vi "PH_AxisGUI_NF2.panel.vi"(0 "object ref":refnum<vi>, 5 "error in (no error)":errorcluster) -> (19 "error out":errorcluster)   [LabVIEW 2014, in "PH_AxisGUI_NF2.lvlib"]
doc: "By this VI a ross relais can be monitored and switched. \n\nThe indicators \"CLOSED\", \"OPEN\" and \"SWITCH STATE\" show the value of the Beckhoff-Tag: blue indicates bad tag status reference problems, darkgreen false and lightgreen on. If everything is working fine, \"CLOSED\" and \"SWITCH STATE\" should show the same value, while \"OPEN\" has the opposite value. \n\nThe oval button switches the ross relais. It should be in the same state as the \"SWITCH STATE\" indicator. \n\n\"EXIT\" closes the front panel (GUI), while \"Delete Instance\" disconnects and removes the instance from the PCS.\n\nThis VI has no machine safety relevant logig: there is neither a check of internal conclict nor with other objects, for example conflict with other ross relais. Therefore it must be handled with care and should be operated by well educated operators only. It is forseen exclusively for direct operating and testing of the system. \n\nLicense Agreement for this software:\n\nCopyright (C)\nGesellschaft für Schwerionenforschung, GSI\nPlanckstr. 1\n64291 Darmstadt\nGermany\n\nContact: D.Beck@gsi.de \n\nThis program is free software; you can redistribute it and/or modify it under the terms of the GNU General Public License as published by the Free Software Foundation; either version 2 of the license, or (at your option) any later version.\n\nThis program is distributed in the hope that it will be useful, but WITHOUT ANYW ARRANTY; without even the implied warranty of MERCHANTABILITY or FITNESS FOR A PARTICULAR PURPOSE. See the GNU General License for more details (http://www.gnu.org).\n\nGesellschaft für Schwerionenforschung, GSI\nPlanckstr. 1, 64291 Darmstadt, Germany\nFor all questions and ideas contact: M.Richter@gsi.de, H.Brand@gsi.de or D.Beck@gsi.de.\nLast update: 18-DEC-2002"
uses:
  PH_AxisGUI_NF2.lvlib
  PH_Common/PH_Common.lvlib
  CSMotion/NF87XX/NF87XX.lvlib
  CSCore/CSSystem/CSSystemLib/CSSystemLib.lvlib
  PH_Class/PH_Class.lvlib
panel:
  in  "DOWN":bool caption="? Steps"
  in  "UP":bool caption="? Steps"
  in  "LEFT":bool caption="? Steps"
  in  "RIGHT":bool caption="? Steps"
  in  "Width Axis 2":i32
  in  "Width Axis 1":i32
  out "Instance Status":u32(colorbox)
  in  "Emergeny Stop":bool
  in  "Delete":bool
  # "PCS"
  # "3.40"
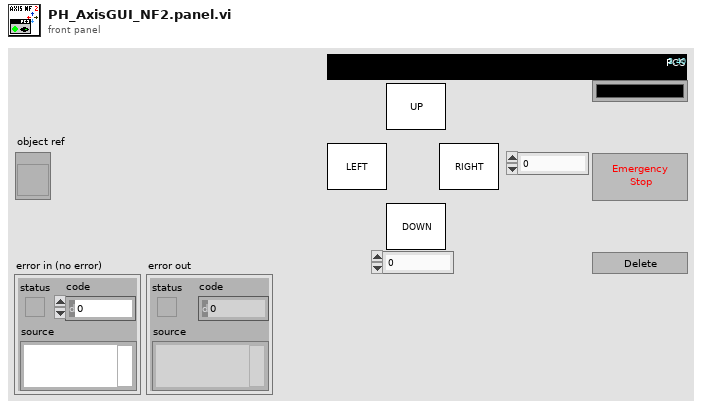
[diagram p1: front panel]
types:
  T1 = typedef "PH_AxisGUI_NF2.lvlib/PH_AxisGUI_NF2.i attribute.ctl" = cluster{"GUI Refs":cluster{"Delete":refnum<vi>, "Instance Status":refnum<vi>, "Width Axis 1":refnum<vi>, "Width Axis 2":refnum<vi>}, "Instance":string, "System":string, "Width Axis 1":i32, "Width Axis 2":i32, "Sign Change Axis 1":bool, "Sign Change Axis 2":bool, "Motor Axis 1":i32, "Motor Axis 2":i32}
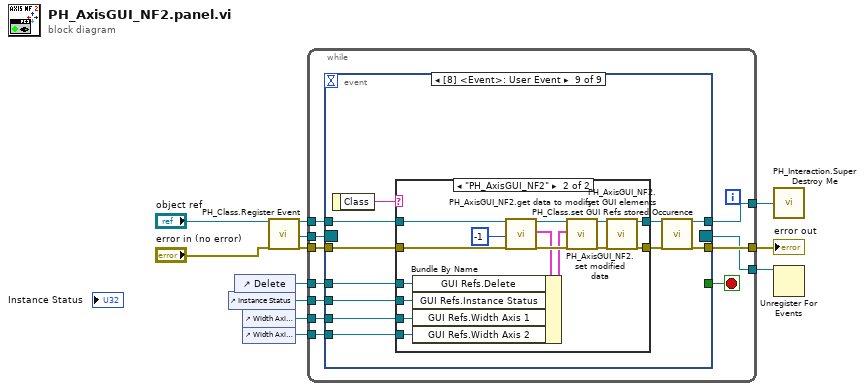
[diagram p0: block diagram]
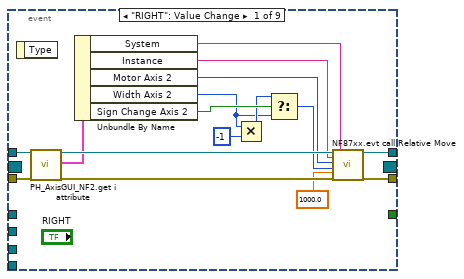
[diagram p2: hidden frame]
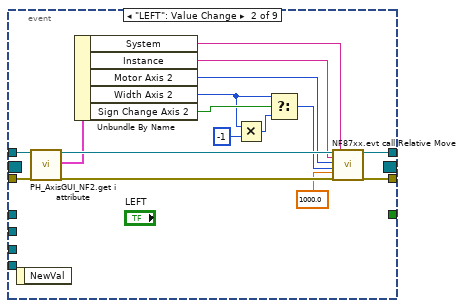
[diagram p3: hidden frame]
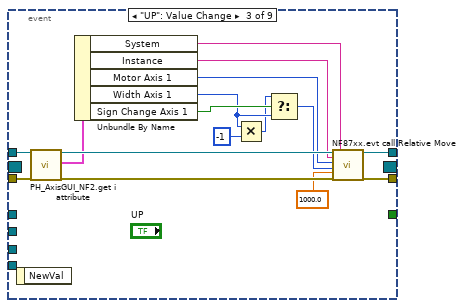
[diagram p4: hidden frame]
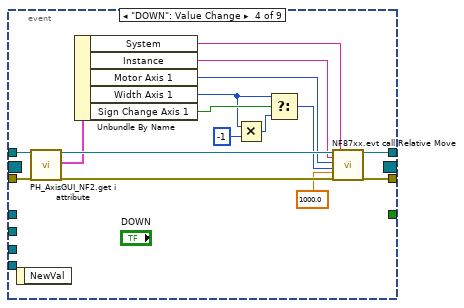
[diagram p5: hidden frame]
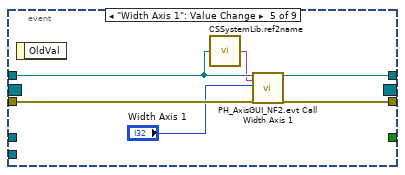
[diagram p6: hidden frame]
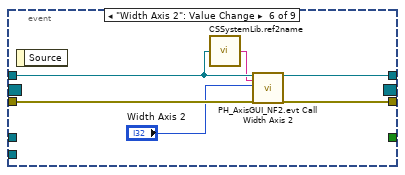
[diagram p7: hidden frame]
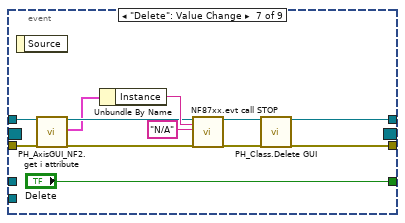
[diagram p8: hidden frame]
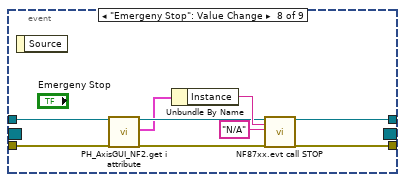
[diagram p9: hidden frame]
diagram:
  n1 = control-ref of="Instance Status"() -> (w3:refnum<vi>)
  n2 = control-ref of="Delete"() -> (w4:refnum<vi>)
  n3 = control-ref of="Width Axis 1"() -> (w2:refnum<vi>)
  n4 = control-ref of="Width Axis 2"() -> (w1:refnum<vi>)
  n5 = call "PH_Class.Register Event.vi"("i ref in"="object ref", "error in (no error)"="error in (no error)") -> ("i ref out"=w10:refnum<vi>, "Event Registration Refnum"=w8:refnum<event-registration>, "error out"=w9:errorcluster)  [unwired: 15 in]
  n6 = while {
    tunnel: w10 -> [w20]
    tunnel: [w19] -> w11
    tunnel: w9 -> [w22]
    tunnel: [w21] -> w12
    tunnel: w8 -> [w18]
    tunnel: [w17] -> w7
    tunnel: w4 -> [w16]
    tunnel: w3 -> [w15]
    tunnel: w2 -> [w14]
    tunnel: w1 -> [w13]
    stop <- w23 stop-if-true
    n7 = event shown="[8] <Event>: User Event" {
      selector: w18 -> [_ _ _ _ _ _ _ _ _]
      dyn-events: [_ _ _ _ _ _ _ _ _] -> w17
      timeout: _ -> [_ _ _ _ _ _ _ _ _]
      tunnel: [_ _ _ _ _ _ "Delete" _ _] -> w23
      tunnel: w20 -> [w37 w53 w69 w85 w89 w96 w106 w116 w131]
      tunnel: w22 -> [w35 w51 w67 w83 w92 w98 w104 w115 w128]
      tunnel: [w38 w54 w70 w86 w91 w97 w100 w112 w126] -> w21
      tunnel: [w39 w55 w71 w87 w93 w99 w101 w113 w129] -> w19
      tunnel: w16 -> [_ _ _ _ _ _ _ _ w124]
      tunnel: w15 -> [_ _ _ _ _ _ _ _ w123]
      tunnel: w14 -> [_ _ _ _ _ _ _ _ w122]
      tunnel: w13 -> [_ _ _ _ _ _ _ _ w121]
      event "RIGHT": Value Change {
        n8 = event-data() -> ()  [unwired: 1 in, 1 out]
        n9 = call "PH_AxisGUI_NF2.get i attribute.vi"("i ref in"=w37, "error in (no error)"=w35) -> ("i ref out"=w36:refnum<vi>, "i attribute"=w33:T1, "error out"=w34:errorcluster)  [unwired: 15 in]
        n10 = Unbundle By Name(w33) -> ("System"=w32:string, "Instance"=w31:string, "Motor Axis 2"=w29:i32, "Width Axis 2"=w24:i32, "Sign Change Axis 2"=w28:bool)
        n11 = Multiply(x=w24, y=-1) -> (x*y=w25:i32)
        n12 = Select(t=w25, s=w28, f=w24) -> (s? t:f=w27:i32)
        n13 = call "NF87xx.evt call Relative Move.vi"("i ref in"=w36, "Instance"=w31, "Motor (0, 1 or 2)"=w29, "steps"=w27, "velocity (10 .. 2000)"=1000.0, "error in (no error)"=w34, "System"=w32) -> ("i ref out"=w39:refnum<vi>, "error out"=w38:errorcluster)  [unwired: 11 in]
      }
      event "LEFT": Value Change {
        n14 = event-data() -> ()  [unwired: 1 in, 1 out]
        n15 = call "PH_AxisGUI_NF2.get i attribute.vi"("i ref in"=w53, "error in (no error)"=w51) -> ("i ref out"=w52:refnum<vi>, "i attribute"=w49:T1, "error out"=w50:errorcluster)  [unwired: 15 in]
        n16 = Unbundle By Name(w49) -> ("System"=w48:string, "Instance"=w47:string, "Motor Axis 2"=w45:i32, "Width Axis 2"=w42:i32, "Sign Change Axis 2"=w44:bool)
        n17 = Multiply(x=w42, y=-1) -> (x*y=w41:i32)
        n18 = Select(t=w42, s=w44, f=w41) -> (s? t:f=w43:i32)
        n19 = call "NF87xx.evt call Relative Move.vi"("i ref in"=w52, "Instance"=w47, "Motor (0, 1 or 2)"=w45, "steps"=w43, "velocity (10 .. 2000)"=1000.0, "error in (no error)"=w50, "System"=w48) -> ("i ref out"=w55:refnum<vi>, "error out"=w54:errorcluster)  [unwired: 11 in]
      }
      event "UP": Value Change {
        n20 = event-data() -> ()  [unwired: 1 in, 1 out]
        n21 = call "PH_AxisGUI_NF2.get i attribute.vi"("i ref in"=w69, "error in (no error)"=w67) -> ("i ref out"=w68:refnum<vi>, "i attribute"=w65:T1, "error out"=w66:errorcluster)  [unwired: 15 in]
        n22 = Unbundle By Name(w65) -> ("System"=w64:string, "Instance"=w63:string, "Motor Axis 1"=w61:i32, "Width Axis 1"=w57:i32, "Sign Change Axis 1"=w60:bool)
        n23 = Multiply(x=w57, y=-1) -> (x*y=w56:i32)
        n24 = Select(t=w56, s=w60, f=w57) -> (s? t:f=w59:i32)
        n25 = call "NF87xx.evt call Relative Move.vi"("i ref in"=w68, "Instance"=w63, "Motor (0, 1 or 2)"=w61, "steps"=w59, "velocity (10 .. 2000)"=1000.0, "error in (no error)"=w66, "System"=w64) -> ("i ref out"=w71:refnum<vi>, "error out"=w70:errorcluster)  [unwired: 11 in]
      }
      event "DOWN": Value Change {
        n26 = event-data() -> ()  [unwired: 1 in, 1 out]
        n27 = call "PH_AxisGUI_NF2.get i attribute.vi"("i ref in"=w85, "error in (no error)"=w83) -> ("i ref out"=w84:refnum<vi>, "i attribute"=w81:T1, "error out"=w82:errorcluster)  [unwired: 15 in]
        n28 = Unbundle By Name(w81) -> ("System"=w80:string, "Instance"=w79:string, "Motor Axis 1"=w77:i32, "Width Axis 1"=w73:i32, "Sign Change Axis 1"=w76:bool)
        n29 = Multiply(x=w73, y=-1) -> (x*y=w72:i32)
        n30 = Select(t=w73, s=w76, f=w72) -> (s? t:f=w75:i32)
        n31 = call "NF87xx.evt call Relative Move.vi"("i ref in"=w84, "Instance"=w79, "Motor (0, 1 or 2)"=w77, "steps"=w75, "velocity (10 .. 2000)"=1000.0, "error in (no error)"=w82, "System"=w80) -> ("i ref out"=w87:refnum<vi>, "error out"=w86:errorcluster)  [unwired: 11 in]
      }
      event "Width Axis 1": Value Change {
        n32 = event-data() -> ()  [unwired: 1 in, 1 out]
        n33 = call "CSSystemLib.ref2name.vi"("obj refnum"=w89) -> ("name"=w88:string)
        n34 = call "PH_AxisGUI_NF2.evt Call Width Axis 1.vi"("i ref in"=w89, "NF GUI 2 instance"=w88, "Width Axis 1"="Width Axis 1", "error in"=w92) -> ("i ref out"=w93:refnum<vi>, "error out"=w91:errorcluster)  [unwired: 14 in]
      }
      event "Width Axis 2": Value Change {
        n35 = event-data() -> ()  [unwired: 1 in, 1 out]
        n36 = call "CSSystemLib.ref2name.vi"("obj refnum"=w96) -> ("name"=w95:string)
        n37 = call "PH_AxisGUI_NF2.evt Call Width Axis 2.vi"("i ref in"=w96, "NF GUI 2 instance"=w95, "Width Axis 1"="Width Axis 2", "error in"=w98) -> ("i ref out"=w99:refnum<vi>, "error out"=w97:errorcluster)  [unwired: 14 in]
      }
      event "Delete": Value Change {
        n38 = event-data() -> ()  [unwired: 1 in, 1 out]
        n39 = call "PH_AxisGUI_NF2.get i attribute.vi"("i ref in"=w106, "error in (no error)"=w104) -> ("i ref out"=w108:refnum<vi>, "i attribute"=w103:T1, "error out"=w107:errorcluster)  [unwired: 15 in]
        n40 = Unbundle By Name(w103) -> ("Instance"=w110:string)
        n41 = call "NF87xx.evt call STOP.vi"("i ref in"=w108, "Instance"=w110, "System (N/A)"="N/A", "error in (no error)"=w107) -> ("i ref out"=w105:refnum<vi>, "error out"=w102:errorcluster)  [unwired: 14 in]
        n42 = call "PH_Class.Delete GUI.vi"("VI in"=w105, "error in (no error)"=w102) -> ("VI out"=w101:refnum<vi>, "error out"=w100:errorcluster)  [unwired: 16 in]
      }
      event "Emergeny Stop": Value Change {
        n43 = event-data() -> ()  [unwired: 1 in, 1 out]
        n44 = call "PH_AxisGUI_NF2.get i attribute.vi"("i ref in"=w116, "error in (no error)"=w115) -> ("i ref out"=w118:refnum<vi>, "i attribute"=w114:T1, "error out"=w117:errorcluster)  [unwired: 15 in]
        n45 = Unbundle By Name(w114) -> ("Instance"=w120:string)
        n46 = call "NF87xx.evt call STOP.vi"("i ref in"=w118, "Instance"=w120, "System (N/A)"="N/A", "error in (no error)"=w117) -> ("i ref out"=w113:refnum<vi>, "error out"=w112:errorcluster)  [unwired: 14 in]
      }
      event User Event {
        n47 = event-data() -> ("Class"=w125:string)  [unwired: 1 in]
        n48 = case shown="\"PH_AxisGUI_NF2\"" w125 {
          tunnel: w131 -> [w133 w143]
          tunnel: [w133 w141] -> w130
          tunnel: w128 -> [w132 w140]
          tunnel: [w132 w138] -> w127
          tunnel: w124 -> [_ w137]
          tunnel: w123 -> [_ w136]
          tunnel: w122 -> [_ w135]
          tunnel: w121 -> [_ w134]
          frame Default {
          }
          frame "PH_AxisGUI_NF2" {
            n49 = call "PH_AxisGUI_NF2.get data to modify.vi"("i ref in"=w143, "ms timeout (10000)"=-1, "error in (no error)"=w140) -> ("i ref out"=w148:refnum<vi>, "i attribute"=w145:T1, "error out"=w147:errorcluster)  [unwired: 13 in, 1 out]
            n50 = Bundle By Name(cluster=w145, "GUI Refs.Delete"=w137, "GUI Refs.Instance Status"=w136, "GUI Refs.Width Axis 1"=w135, "GUI Refs.Width Axis 2"=w134) -> (w144:T1)
            n51 = call "PH_AxisGUI_NF2.set modified data.vi"("i ref in"=w148, "i attribute"=w144, "error in (no error)"=w147) -> ("i ref out"=w142:refnum<vi>, "error out"=w139:errorcluster)  [unwired: 15 in]
            n52 = call "PH_AxisGUI_NF2.set GUI elements.vi"("i ref in"=w142, "error in (no error)"=w139) -> ("i ref out"=w141:refnum<vi>, "error out"=w138:errorcluster)  [unwired: 16 in]
          }
        }
        n53 = call "PH_Class.set GUI Refs stored Occurence.vi"("i ref in"=w130, "error in (no error)"=w127) -> ("i ref out"=w129:refnum<vi>, "error out"=w126:errorcluster)  [unwired: 16 in]
      }
    }
  }
  "error out" <- w12
  n54 = call "PH_Interaction.Super Destroy Me.vi"("i ref out"=w11) -> ()
  n55 = Unregister For Events(event registration refnum=w7) -> ()  [unwired: 1 in, 1 out]
